vi "Set Bytes Progress by val.vi"(8 "error in (no error)":errorcluster, 10 "bytes downloaded":i64, 11 "HTTP GET Async in":refnum<class "GET Async.lvclass">) -> (0 "error out":errorcluster, 3 "HTTP GET Async out":refnum<class "GET Async.lvclass">)   [LabVIEW 2019, in "HTTP Client Extensions.lvlib" / "GET Async.lvclass"]
uses:
  GET Async.lvclass
  GET Async.lvclass/GET Async.ctl
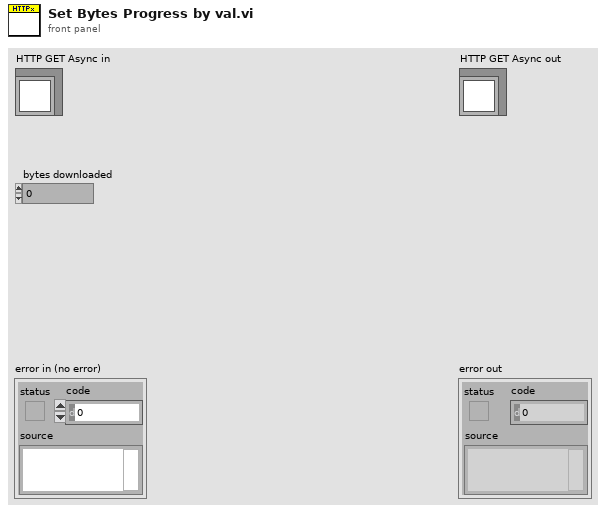
[diagram p1: front panel]
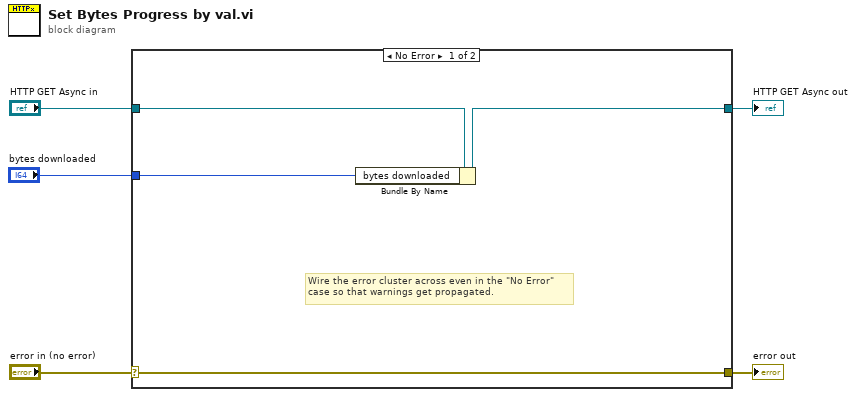
[diagram p0: block diagram]
diagram:
  n1 = case shown="No Error" "error in (no error)" {
    selector: "error in (no error)" -> [w9 w11]
    tunnel: [w9 w11] -> w4
    tunnel: [w7 w10] -> w2
    tunnel: "HTTP GET Async in" -> [w6 w10]
    tunnel: "bytes downloaded" -> [w8 _]
    frame No Error {
      # "Wire the error cluster across even in the \"No Error\"\ncase so that warnings get propagated."
      n2 = Bundle By Name(cluster=w6, "bytes downloaded"=w8) -> (w7:refnum<class "GET Async.lvclass">)
    }
    frame Error {
    }
  }
  "error out" <- w4
  "HTTP GET Async out" <- w2
